vi "UTIL_Add string element to queue v1_0_0.vi"(7 "Flush (f)":bool, 8 "error in (no error)":errorcluster, 9 "Queue position":enum16{"top", "bottom"}(ring)=enum."bottom", 10 "enqueue string":string, 11 "Queue in":refnum<queue>) -> (0 "error out":errorcluster, 3 "Queue out":refnum<queue>)   [LabVIEW 2009]
doc: "UTIL_Add string element to queue v1_0_0.vi\n\nIf flush queue first boolean is true it revoves any existing queue elements from the queue array. If false, Items already existing on the queue array will remain.\n\nThe item that exists in the enqueue string control is then added to either the top or bottom of the queue depending on the Queue position control\n\nEdited 2007 by\nDave Hawley\nWGC\n970-962-7484"
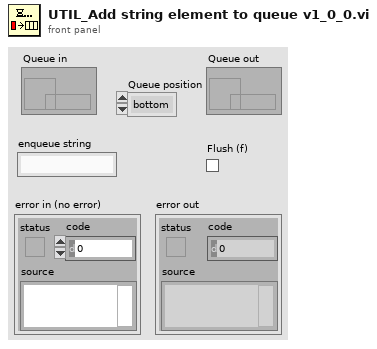
[diagram p1: front panel]
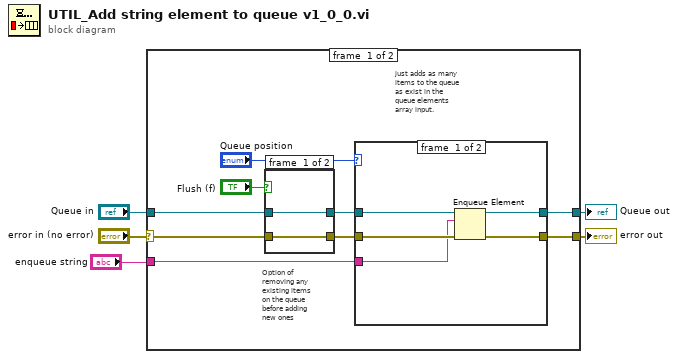
[diagram p0: block diagram]
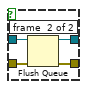
[diagram p2: hidden frame]
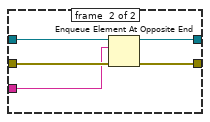
[diagram p3: hidden frame]
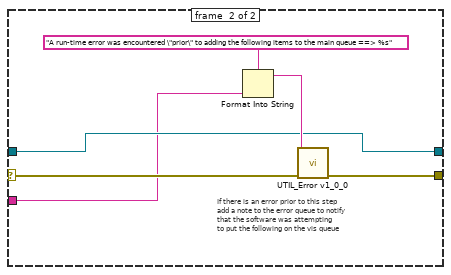
[diagram p4: hidden frame]
diagram:
  n1 = case shown="No Error" "error in (no error)" {
    selector: "error in (no error)" -> [w8 w36]
    tunnel: "Queue in" -> [w14 w33]
    tunnel: [w13 w35] -> w4
    tunnel: "enqueue string" -> [w7 w31]
    tunnel: [w6 w33] -> w2
    frame #0 {
      # "just adds as many\nitems to the queue\nas exist in the\nqueue elements\narray input."
      # "Option of \nremoving any\nexisting items\non the queue\nbefore adding \nnew ones"
      n2 = case shown="True" "Flush (f)" {
        tunnel: w8 -> [w15 w20]
        tunnel: [w15 w19] -> w10
        tunnel: [w16 w18] -> w9
        tunnel: w14 -> [w16 w17]
        frame #0 {
        }
        frame #1 {
          n3 = Flush Queue(queue=w17, error in (no error)=w20) -> (queue out=w18:refnum<queue>, error out=w19:errorcluster)  [unwired: 1 out]
        }
      }
      n4 = case shown="\"bottom\"" "Queue position" {
        tunnel: w9 -> [w25 w30]
        tunnel: [w24 w29] -> w6
        tunnel: [w23 w28] -> w13
        tunnel: w10 -> [w22 w27]
        tunnel: w7 -> [w21 w26]
        frame #0 {
          n5 = Enqueue Element(queue=w25, element=w21, error in (no error)=w22) -> (queue out=w24:refnum<queue>, error out=w23:errorcluster)  [unwired: 2 out]
        }
        frame #1 {
          n6 = Enqueue Element At Opposite End(queue=w30, element=w26, error in (no error)=w27) -> (queue out=w29:refnum<queue>, error out=w28:errorcluster)  [unwired: 2 out]
        }
      }
    }
    frame #1 {
      # "If there is an error prior to this step\nadd a note to the error queue to notify\nthat the software was attempting\nto put the following on the vis queue"
      n7 = Format Into String(format string="A run-time error was encountered \"prior\" to adding the following items to the main queue ==> %s", w31) -> (resulting string=w34:string)  [unwired: 2 in, 1 out]
      n8 = call "UTIL_Error v1_0_0.vi"("error in (no error)"=w36, "State"=w34) -> ("error out"=w35:errorcluster)  [unwired: 1 in, 8 out]
    }
  }
  "error out" <- w4
  "Queue out" <- w2
